vi "Set Server gRPC UEs.vi"(10 "Server gRPC UEs":T1, 11 "OOP Server in":refnum<class "ctet_smu.lvclass">) -> (3 "OOP Server out":refnum<class "ctet_smu.lvclass">)   [LabVIEW 2019, in "ctet_smu.lvlib" / "ctet_smu.lvclass"]
uses:
  ctet_smu.lvclass
  typeDefs/Server gRPC UEs.ctl
  gRPC lvSupport/Server API/typeDefs/gRPCId Cluster.ctl
  gRPC lvSupport/Server API/typeDefs/grpcId.ctl
  ctet_smu.lvclass/ctet_smu.ctl
  gRPC lvSupport/gprc-lvsupport.lvlib
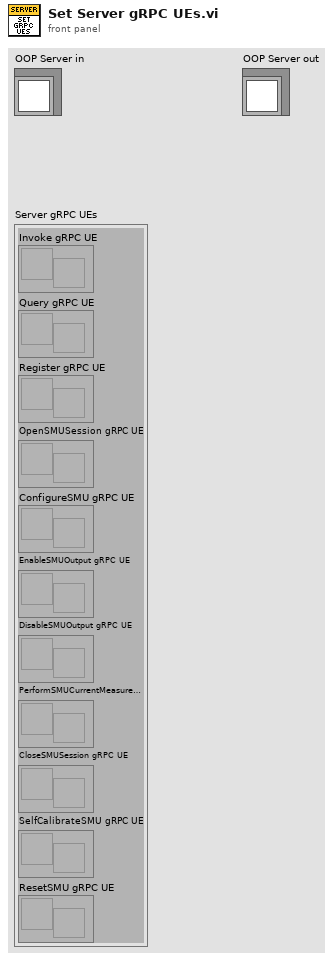
[diagram p1: front panel]
types:
  T1 = typedef "ctet_smu.lvlib/ctet_smu.lvclass/Server gRPC UEs.ctl" = cluster{"Invoke gRPC UE":refnum<user-event>, "Query gRPC UE":refnum<user-event>, "Register gRPC UE":refnum<user-event>, "OpenSMUSession gRPC UE":refnum<user-event>, "ConfigureSMU gRPC UE":refnum<user-event>, "EnableSMUOutput gRPC UE":refnum<user-event>, "DisableSMUOutput gRPC UE":refnum<user-event>, "PerformSMUCurrentMeasurement gRPC UE":refnum<user-event>, "CloseSMUSession gRPC UE":refnum<user-event>, "SelfCalibrateSMU gRPC UE":refnum<user-event>, "ResetSMU gRPC UE":refnum<user-event>}
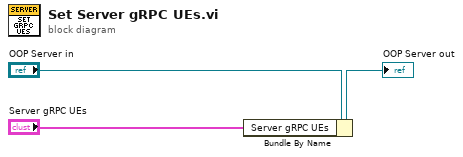
[diagram p0: block diagram]
diagram:
  n1 = Bundle By Name(cluster="OOP Server in", "Server gRPC UEs"="Server gRPC UEs") -> (→"OOP Server out":refnum<class "ctet_smu.lvclass">)
